vi "Send CCD Setup.vi"(8 "error in (no error)":errorcluster, 11 "RxTx in":refnum<class "RxTx.lvclass">) -> (0 "error out":errorcluster, 3 "RxTx out":refnum<class "RxTx.lvclass">)   [LabVIEW 2018]
uses:
  RxTx.lvclass
  Interface/Interface.lvclass
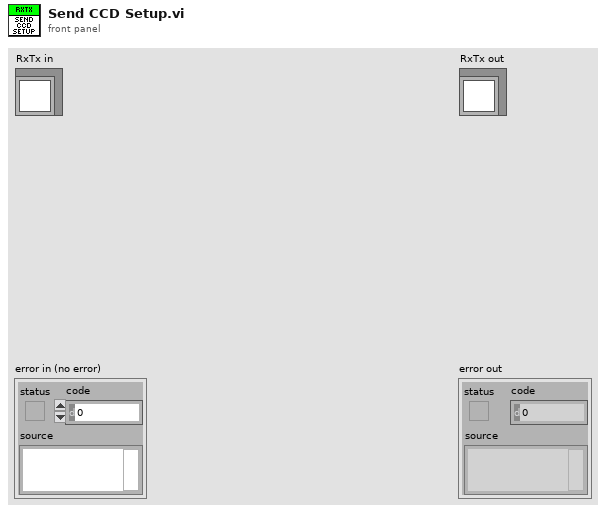
[diagram p1: front panel]
types:
  T1 = cluster{"PREAMP":u16, "READOUT_RATE":u16, "EM_GAIN":u16, "VBIN":u16, "INITIAL_LINE":u16, "INITIAL_COLUMN":u16, "FINAL_LINE":u16, "FINAL_COLUMN":u16, "TRIGGER_MODE":u16, "HBIN":u16, "SHUTTER_TTL":u16, "SHUTTER_MODE":u16, "SHUTTER_OPENING_TIME":u16, "SHUTTER_CLOSING_TIME":u16, "VERTICAL_SHIFT_SPEED":u16, "READ_MODE":u16, "FRAME_TRANSFER":bool, "VERTICAL_CLOCK_VOLTAGE":u16, "ACQUISITION_MODE":u16, "AD_CHANNEL":u16, "EM_MODE":u16}
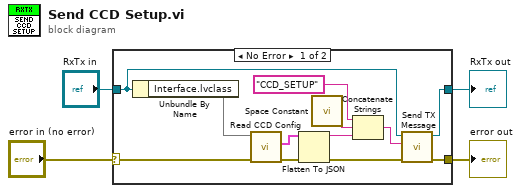
[diagram p0: block diagram]
diagram:
  n1 = case shown="No Error" "error in (no error)" {
    selector: "error in (no error)" -> [w9 w18]
    tunnel: [w13 w18] -> w2
    tunnel: [w14 w17] -> w1
    tunnel: "RxTx in" -> [w15 w17]
    frame No Error {
      n2 = Unbundle By Name(w15) -> ("Interface.lvclass"=w10)
      n3 = call "Read CCD Config.vi"("error in (no error)"=w9, "Interface in"=w10) -> ("error out"=w8:errorcluster, "CCD Config"=w5:T1)  [unwired: 7 in, 1 out]
      n4 = Flatten To JSON(anything=w5, error in (no error)=w8) -> (JSON string=w6:string, 11:w7:errorcluster)  [unwired: 1 in]
      n5 = call <vilib>:"Space Constant.vi"() -> ("String"=w12:string)
      n6 = Concatenate Strings("CCD_SETUP", w12, w6) -> (w16:string)
      n7 = call "Send TX Message.vi"("error in (no error)"=w7, "element"=w16, "RxTx in"=w15) -> ("error out"=w13:errorcluster, "RxTx out"=w14:refnum<class "RxTx.lvclass">)  [unwired: 7 in]
    }
    frame Error {
    }
  }
  "error out" <- w2
  "RxTx out" <- w1
